vi "VDCreateDiagramImage.vi"(10 "VI path":path) -> (2 "image data":T1)   [LabVIEW 2013, in "VIDiagram.lvlib"]
uses:
  <vilib>/picture/picture.llb/imagedata.ctl
  <vilib>/picture/picture.llb/Draw True-Color Pixmap.vi
  VIDiagram.lvlib
panel:
  out "new picture":picture
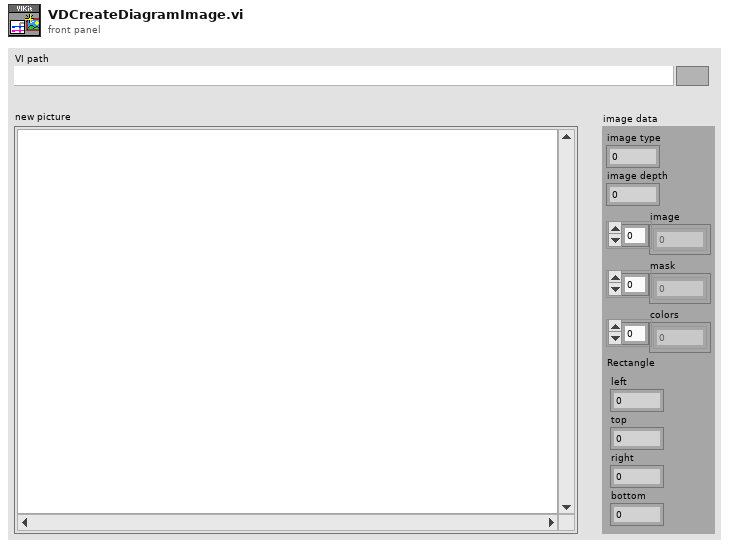
[diagram p1: front panel]
types:
  T1 = typedef "imagedata.ctl" = cluster{"image type":i32, "image depth":i32, "image":u8[], "mask":u8[], "colors":u32[], "Rectangle":cluster{"left":i16, "top":i16, "right":i16, "bottom":i16}}
  T2 = cluster{"left":i16, "top":i16, "right":i16, "bottom":i16}
  T3 = enum32{"Solid", "Dash", "Dot", "DashDot", "DashDotDot"}
  T4 = cluster{"Width":u16, "Style":enum32{"Solid", "Dash", "Dot", "DashDot", "DashDotDot"}}
  T5 = cluster{"Font Name:":string, "Size":i16, "Strikeout?":bool, "Italic?":bool, "Underline?":bool, "Outline?":bool, "Shadow?":bool, "Bold?":bool}
  T6 = enum16{"User-specified Font", "Application Font", "System Font", "Dialog Font"}
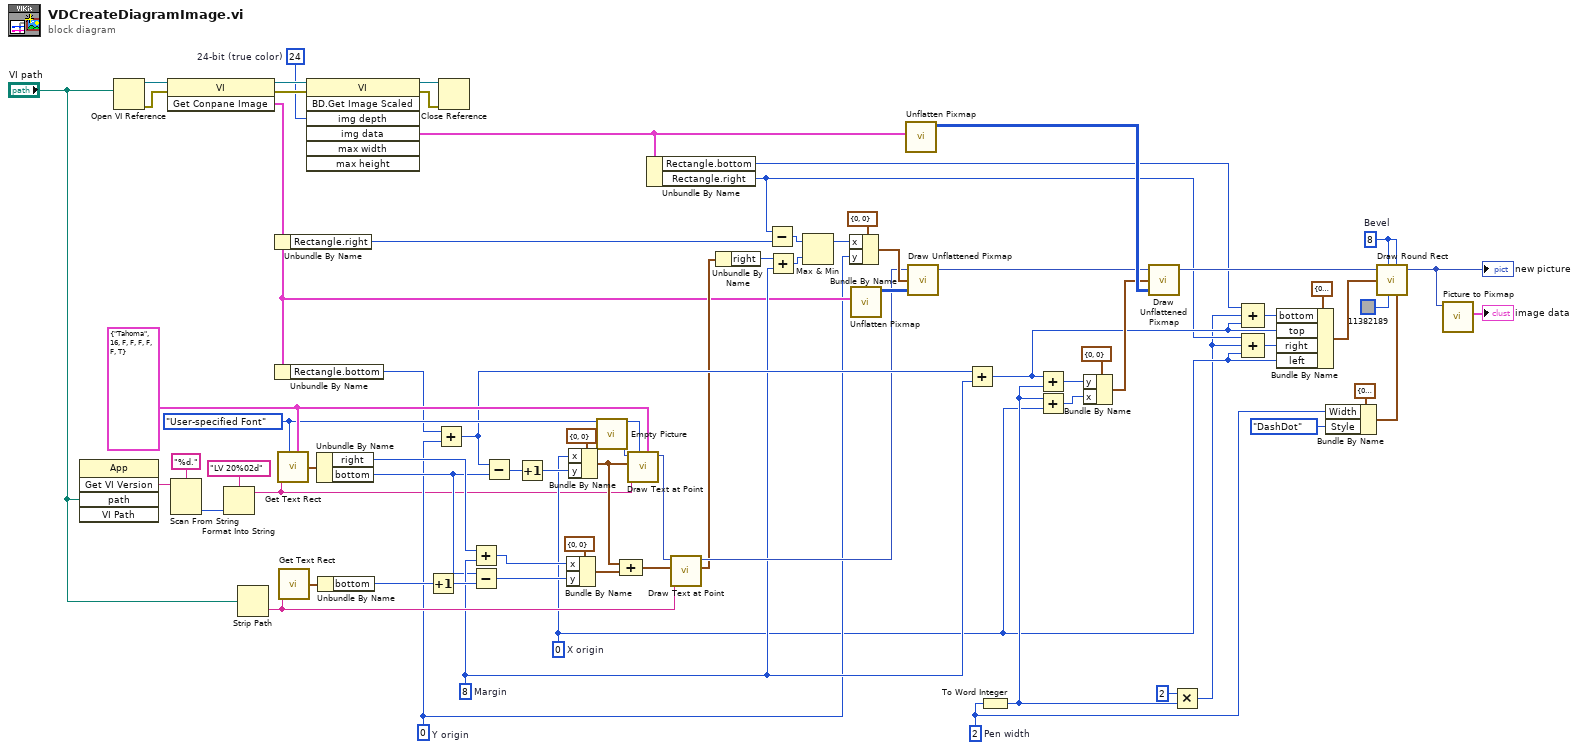
[diagram p0: block diagram]
diagram:
  w31 = u16 2  # Pen width
  w42 = i16 8  # Bevel
  w20 = i16 0  # Y origin
  w35 = i16 8  # Margin
  w15 = i16 0  # X origin
  w53 = T5 {"Font Name:"="Tahoma", "Size"=16, "Strikeout?"=FALSE, "Italic?"=FALSE, "Underline?"=FALSE, "Outline?"=FALSE, "Shadow?"=FALSE, "Bold?"=TRUE} ("[user-specified font]")
  w52 = T6."User-specified Font" ("desired font(Application)")
  w69 = 24  # 24-bit (true color)
  n1 = invoke class="App" method="Get VI Version"("path"="VI path") -> ("GetVIVers"=w6:string)  [unwired: 4 in, 4 out]
  n2 = Open VI Reference(vi path="VI path") -> (vi reference=w74:refnum<vi>, error out=w75:errorcluster)  [unwired: 5 in]
  n3 = invoke class="VI" method="Get Conpane Image"(reference=w74, error in=w75) -> (reference out=w72:refnum<vi>, error out=w73:errorcluster, "Get Conpane Image"=w28:T1)  [unwired: 1 in]
  n4 = Scan From String(format string="%d.", input string=w6) -> (output 1=w4:i32)  [unwired: 3 in, 3 out]
  n5 = Format Into String(format string="LV 20%02d", w4) -> (resulting string=w3:string)  [unwired: 2 in, 1 out]
  n6 = Strip Path(path="VI path") -> (name=w59:string)  [unwired: 1 out]
  n7 = Unbundle By Name(w28) -> ("Rectangle.right"=w44:i16)
  n8 = Unbundle By Name(w28) -> ("Rectangle.bottom"=w27:i16)
  n9 = call <vilib>:"Get Text Rect.vi"("desired font(Application)"=w52, "text"=w3, "[user-specified font]"=w53) -> ("rect"=w49:T2)  [unwired: 6 in]
  n10 = call <vilib>:"Get Text Rect.vi"("text"=w59) -> ("rect"=w68:T2)  [unwired: 8 in]
  n11 = invoke class="VI" method="BD.Get Image Scaled"(reference=w72, error in=w73, "img depth"=w69) -> (reference out=w71:refnum<vi>, error out=w70:errorcluster, "img data"=w46:T1)  [unwired: 4 in, 4 out]
  n12 = Unbundle By Name(w49) -> ("right"=w61:i16, "bottom"=w29:i16)
  n13 = Unbundle By Name(w68) -> ("bottom"=w67:i16)
  n14 = Increment(x=w67) -> (x+1=w63:i16)
  n15 = Add(x=w27, y=w20) -> (x+y=w47:i16)
  n16 = Close Reference(reference=w71, error in (no error)=w70) -> ()  [unwired: 1 out]
  n17 = Add(x=w61, y=w35) -> (x+y=w62:i16)
  n18 = Subtract(x=w29, y=w63) -> (x-y=w64:i16)
  n19 = Subtract(x=w47, y=w29) -> (x-y=w19:i16)
  n20 = Increment(x=w19) -> (x+1=w18:i16)
  n21 = Bundle By Name(cluster=cluster{"x":i16, "y":i16} {"x"=0, "y"=0} ("origin"), "x"=w62, "y"=w64) -> (w65:cluster{"x":i16, "y":i16})
  n22 = Bundle By Name(cluster=cluster{"x":i16, "y":i16} {"x"=0, "y"=0} ("origin"), "x"=w15, "y"=w18) -> (w43:cluster{"x":i16, "y":i16})
  n23 = call "Empty Picture"() -> ("empty picture"=w26:picture)
  n24 = Compound Arithmetic op=ADD(w43, w65) -> (w60:cluster{"x":i16, "y":i16})
  n25 = call <vilib>:"Draw Text at Point.vi"("[user-specified font]"=w53, "desired font(Application)"=w52, "text"=w3, "origin"=w43, "picture"=w26) -> ("new picture"=w39:picture)  [unwired: 5 in, 1 out]
  n26 = Unbundle By Name(w46) -> ("Rectangle.bottom"=w9:i16, "Rectangle.right"=w12:i16)
  n27 = call <vilib>:"Draw Text at Point.vi"("text"=w59, "origin"=w60, "picture"=w39) -> ("text rect"=w36:T2, "new picture"=w37:picture)  [unwired: 7 in]
  n28 = Unbundle By Name(w36) -> ("right"=w55:i16)
  n29 = Subtract(x=w12, y=w44) -> (x-y=w50:i16)
  n30 = Add(x=w55, y=w35) -> (x+y=w51:i16)
  n31 = Max & Min(x=w50, y=w51) -> (max(x,y)=w45:i16)  [unwired: 1 out]
  n32 = Bundle By Name(cluster=cluster{"x":i16, "y":i16} {"x"=0, "y"=0} ("top left point(0, 0)"), "x"=w45, "y"=w20) -> (w57:cluster{"x":i16, "y":i16})
  n33 = call <vilib>:"Unflatten Pixmap.vi"("image data"=w28) -> ("24-bit pixmap"=w58:u32[][])  [unwired: 4 in, 6 out]
  n34 = call <vilib>:"Unflatten Pixmap.vi"("image data"=w46) -> ("24-bit pixmap"=w48:u32[][])  [unwired: 4 in, 6 out]
  n35 = call-poly <vilib>:"Draw Unflattened Pixmap.vi"("picture"=w37, "top left point(0, 0)"=w57, "data (RGB format)"=w58) -> ("new picture"=w38:picture)  [unwired: 6 in]
  n36 = Add(x=w47, y=w35) -> (x+y=w13:i16)
  n37 = To Word Integer(number=w31) -> (16bit integer=w21:i16)
  n38 = Add(x=w13, y=w21) -> (x+y=w24:i16)
  n39 = Add(x=w21, y=w15) -> (x+y=w23:i16)
  n40 = Bundle By Name(cluster=cluster{"x":i16, "y":i16} {"x"=0, "y"=0} ("top left point(0, 0)"), "y"=w24, "x"=w23) -> (w22:cluster{"x":i16, "y":i16})
  n41 = call-poly <vilib>:"Draw Unflattened Pixmap.vi"("picture"=w38, "top left point(0, 0)"=w22, "data (RGB format)"=w48) -> ("new picture"=w40:picture)  [unwired: 6 in]
  n42 = Multiply(x=i16 2, y=w21) -> (x*y=w11:i16)
  n43 = Compound Arithmetic op=ADD(w9, w11, w13) -> (w14:i16)
  n44 = Compound Arithmetic op=ADD(w12, w11, w15) -> (w16:i16)
  n45 = Bundle By Name(cluster=T2 {"left"=0, "top"=0, "right"=0, "bottom"=0} ("rect"), "bottom"=w14, "top"=w13, "right"=w16, "left"=w15) -> (w10:T2)
  n46 = Bundle By Name(cluster=T4 {"Width"=0, "Style"=enum."Solid"} ("input cluster"), "Width"=w31, "Style"=T3."DashDot") -> (w32:T4)
  n47 = call <vilib>:"Draw Round Rect.vi"("picture"=w40, "oval width"=w42, "rect"=w10, "color(black)"=u32 11382189, "oval height"=w42, "pen"=w32) -> ("new picture"=w2:picture)  [unwired: 3 in]
  "new picture" <- w2
  n48 = call <vilib>:"Picture to Pixmap.vi"("picture"=w2) -> ("image data"=→"image data":T1)  [unwired: 9 in, 1 out]
